vi "Update.vi"(8 "error in (no error)":errorcluster, 10 "Audio Block In":dbl[][](array[numeric]), 11 "Effect Unit in":refnum<class "Effect Unit.lvclass">) -> (0 "error out":errorcluster, 2 "Audio Block Out":dbl[][](array[numeric]), 3 "Effect Unit out":refnum<class "Effect Unit.lvclass">)   [LabVIEW 2019, in "Effect Unit.lvclass"]
uses:
  Effect Unit.lvclass
  Effect Unit.lvclass/Effect Unit.ctl
  Plugin Interfaces/Effect Interface/Effect Interface.lvlibp/Plugin Interfaces/Effect Interface/Effect Interface Class/Effect Interface.lvclass
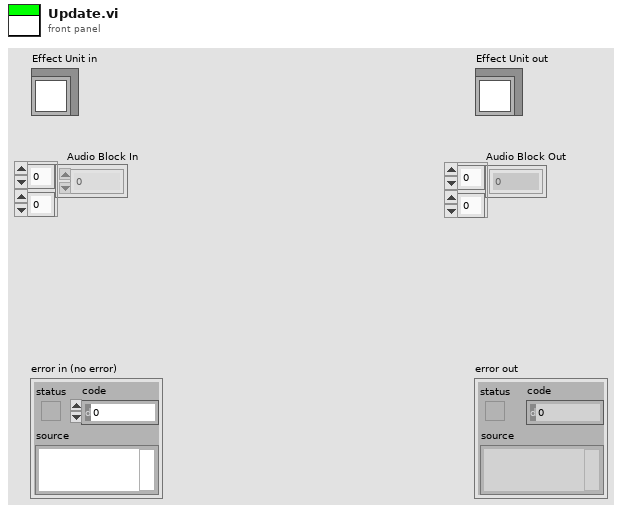
[diagram p1: front panel]
types:
  T1 = typedef "Effect Unit.lvclass/Effect Info.ctl" = cluster{"ID":string, "Message Queue":refnum<queue>, "Effect Interface":refnum<class "Effect Interface.lvclass">}
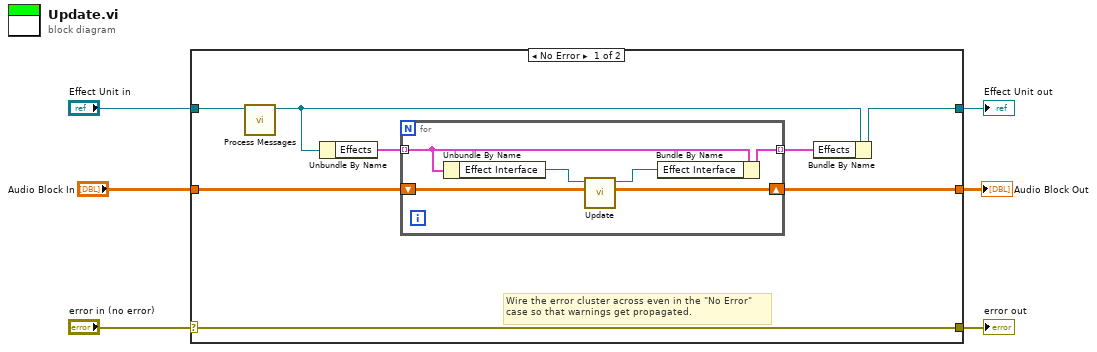
[diagram p0: block diagram]
diagram:
  n1 = case shown="No Error" "error in (no error)" {
    selector: "error in (no error)" -> [w14 w23]
    tunnel: [w14 w23] -> w5
    tunnel: [w9 w22] -> w3
    tunnel: "Effect Unit in" -> [w13 w22]
    tunnel: [w8 w21] -> w2
    tunnel: "Audio Block In" -> [w12 w21]
    frame No Error {
      # "Wire the error cluster across even in the \"No Error\"\ncase so that warnings get propagated."
      n2 = call "Process Messages.vi"("Effect Unit in"=w13) -> ("Effect Unit out"=w10:refnum<class "Effect Unit.lvclass">)  [unwired: 9 in, 1 out]
      n3 = Unbundle By Name(w10) -> ("Effects"=w11:T1[])
      n4 = for {
        shift-right: [w19] -> w8
        shift-left: w12 -> [w20]
        tunnel: w11 -> [w16] mode=indexing
        tunnel: [w15] -> w7 mode=indexing
        n5 = Unbundle By Name(w16) -> ("Effect Interface"=w18:refnum<class "Effect Interface.lvclass">)
        n6 = call-dynamic "Update.vi"("Audio Data In"=w20, "Effect Interface in"=w18) -> ("Audio Data Out"=w19:dbl[][], "Effect Interface out"=w17:refnum<class "Effect Interface.lvclass">)  [unwired: 7 in, 1 out]
        n7 = Bundle By Name(cluster=w16, "Effect Interface"=w17) -> (w15:T1)
      }
      n8 = Bundle By Name(cluster=w10, "Effects"=w7) -> (w9:refnum<class "Effect Unit.lvclass">)
    }
    frame Error {
    }
  }
  "error out" <- w5
  "Effect Unit out" <- w3
  "Audio Block Out" <- w2
